vi "Append to event log.vi"(8 "error in":errorcluster, 10 "Type":string="General", 11 "string":string) -> (0 "error out":errorcluster)   [LabVIEW 2018]
uses:
  CAEN globals.vi
  <vilib>/Utility/file.llb/Write Delimited Spreadsheet (string).vi
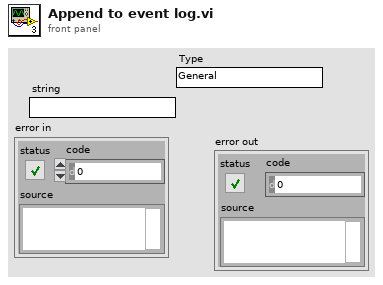
[diagram p1: front panel]
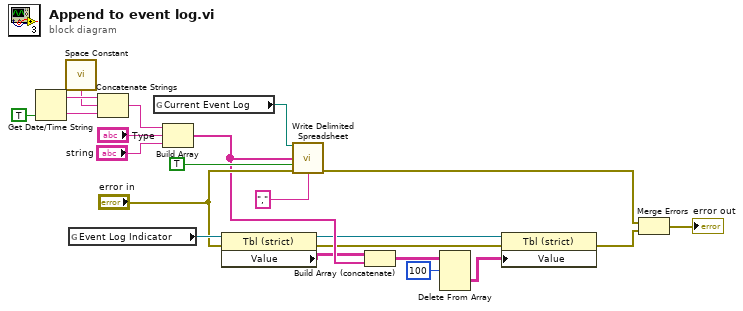
[diagram p0: block diagram]
diagram:
  n1 = Get Date/Time String(want seconds? (F)=TRUE) -> (date string=w17:string, time string=w18:string)  [unwired: 2 in]
  n2 = call <vilib>:"Space Constant.vi"() -> ("String"=w16:string)
  n3 = global read "CAEN globals.vi" "Event Log Indicator"() -> (w12:refnum<vi>)
  n4 = Concatenate Strings(w17, w16, w18) -> (w15:string)
  n5 = global read "CAEN globals.vi" "Current Event Log"() -> (w20:path)
  n6 = Build Array(w15, "Type", "string") -> (w10:string[])
  n7 = property class="Tbl (strict)"(reference=w12, error in="error in") -> (reference out=w7:refnum<vi>, error out=w8:errorcluster, "Value"=w9:string[][])
  n8 = call-poly <vilib>:"Write Delimited Spreadsheet.vi"("file path (dialog if empty)"=w20, "1D data"=w10, "append to file? (new file:F)"=TRUE ("ignore duplicate delimiters? (F=No)"), "error in (no error)"="error in", "delimiter (\\t)"="," ("delimiter (\\t)")) -> ("error out"=w5:errorcluster)  [unwired: 9 in, 1 out]
  n9 = Build Array (concatenate)(w9, w10) -> (w3:string[][])
  n10 = Delete From Array(array=w3, length=100) -> (deleted portion=w2:string[][])  [unwired: 2 in, 1 out]
  n11 = property class="Tbl (strict)"(reference=w7, error in=w8, "Value"=w2) -> (error out=w4:errorcluster)  [unwired: 1 out]
  n12 = Merge Errors(w5, w4) -> (→"error out":errorcluster)
